vi "Scale Can Temp.vi"(11 "Numeric":u16) -> (3 "Double out":dbl)   [LabVIEW 2015]
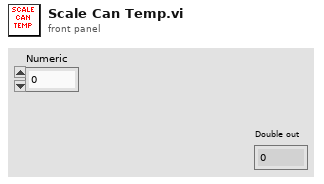
[diagram p1: front panel]
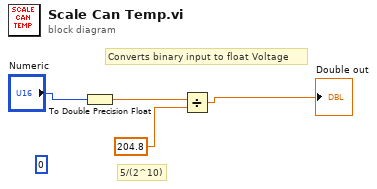
[diagram p0: block diagram]
diagram:
  (unwired) 0
  # "Converts binary input to float Voltage"
  # "5/(2^10)"
  n1 = To Double Precision Float(number="Numeric") -> (double precision float=w2:dbl)
  n2 = Divide(x=w2, y=204.8) -> (x/y=→"Double out":dbl)
